vi "Assert Not Error Code.vi"(5 "Expected":i32, 7 "Message (\"\")":string, 8 "error in (no error)":errorcluster) -> (0 "error out":errorcluster)   [LabVIEW 2017, in "Transparent Assertions.lvlib"]
doc: "Asserts that the error code of <B>error in</B> does not match the expected value. Returns an error if the assertion fails, and optionally appends a custom message to the error."
uses:
  Transparent Assertions.lvlib
  LogicalNot/LogicalNot.lvclass
  ErrorCode/ErrorCode.lvclass
  C:/Users/pasca/Projects/Home/TransparentAssertions/src/Transparent Assertions/Constraints/Constraint/Constraint.lvclass
  UnaryOperator/UnaryOperator.lvclass
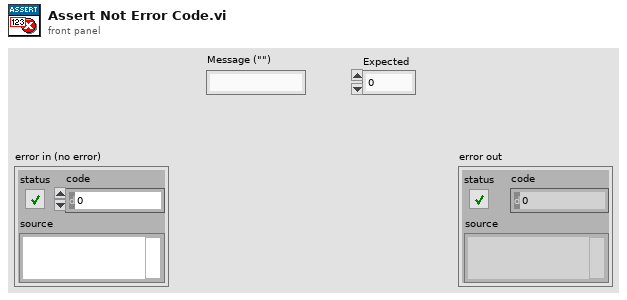
[diagram p1: front panel]
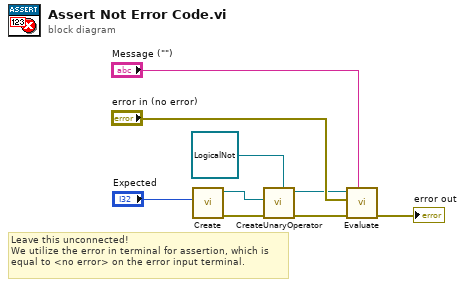
[diagram p0: block diagram]
diagram:
  # "Leave this unconnected!\nWe utilize the error in terminal for assertion, which is\nequal to <no error> on the error input terminal."
  n1 = call "Create.vi"("Expected"="Expected") -> ("error out"=w8:errorcluster, "ErrorCode"=w3:refnum<class "ErrorCode.lvclass">)  [unwired: 9 in]
  n2 = call-dynamic "CreateUnaryOperator.vi"("UnaryOperator In"=refnum<class "LogicalNot.lvclass"> refnum ("Transparent Assertions.lvlib:Constraints.lvlib:LogicalNot.lvclass"), "error in (no error)"=w8, "Constraint"=w3) -> ("error out"=w4:errorcluster, "UnaryOperator"=w2:refnum<class "UnaryOperator.lvclass">)  [unwired: 7 in]
  n3 = call-dynamic "Evaluate.vi"("Message (\"\")"="Message (\"\")", "error in (no error)"=w4, "Actual"="error in (no error)", "Constraint in"=w2) -> ("error out"=→"error out":errorcluster)  [unwired: 6 in, 1 out]
